vi "State_Machine.vi"(8 "error in (no error)":errorcluster caption="entrée d'erreur (pas d'erreur)", 11 "Get_Voltage en entrée":refnum<class "Stop_Blink_Relay.lvclass">) -> (0 "error out":errorcluster caption="sortie d'erreur", 2 "Json_String":string, 3 "Get_Voltage en sortie":refnum<class "Stop_Blink_Relay.lvclass">)   [LabVIEW 2020, in "Library Test.lvlib" / "Stop_Blink_Relay.lvclass"]
uses:
  Stop_Blink_Relay.lvclass
  Commun VI/TypeDef/Variable Printable.ctl
  Commun VI/Library Commun.lvlib
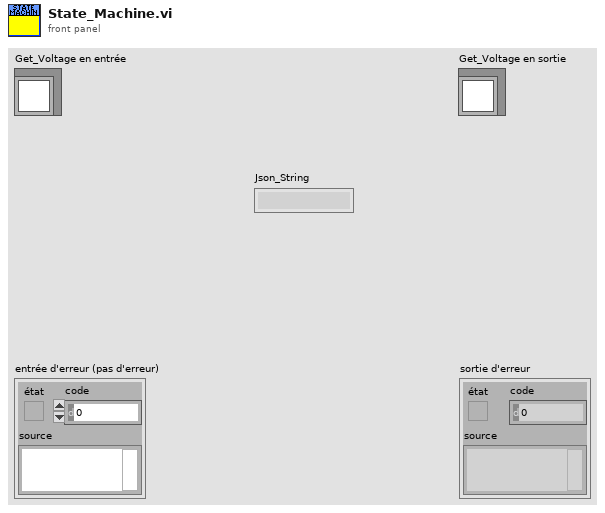
[diagram p1: front panel]
types:
  T1 = typedef "Variable Printable.ctl" = string
  T2 = enum16{"Get Variable", "Get All Variables", "Set Variable", "Delete Variable", "Delete All Variable"}
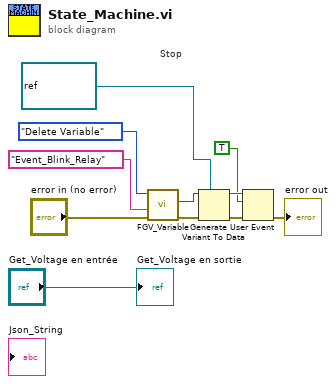
[diagram p0: block diagram]
diagram:
  w5 = refnum<user-event> refnum  # Stop
  n1 = call "FGV_Variable.vi"("error in (no error)"="error in (no error)", "Variable"=T1 "Event_Blink_Relay", "Function"=T2."Delete Variable") -> ("error out"=w4:errorcluster, "Data Out"=w8:variant)  [unwired: 6 in, 1 out]
  n2 = Variant To Data(error in=w4, type=w5, Variant=w8) -> (data=w6:refnum<user-event>, error out=w7:errorcluster)
  n3 = Generate User Event(user event=w6, event data cluster=TRUE ("données d'événement"), error in=w7) -> (error out=→"error out":errorcluster)  [unwired: 1 in, 1 out]
  "Get_Voltage en sortie" <- "Get_Voltage en entrée"
